vi "Settings.vi"(8 "error in (no error)":errorcluster, 9 "Gantry Region":i32=1, 11 "Assembly Tray In":refnum<class "Assembly Tray.lvclass">) -> (0 "error out":errorcluster, 3 "Assembly Tray Out":refnum<class "Assembly Tray.lvclass">)   [LabVIEW 2020, in "Assembly Tray.lvclass"]
uses:
  Assembly Tray.lvclass
panel:
  in  "Component Thickness":dbl=2.0 format="%#_13g"
  in  "Submit":bool
  in  "Position Number":i32=1
  in  "Tray Number":i32=1
  # "Assembly Tray"
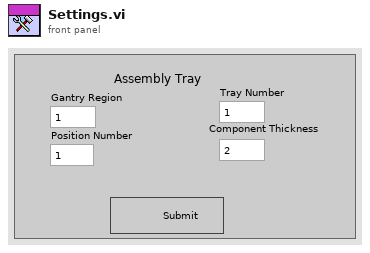
[diagram p1: front panel]
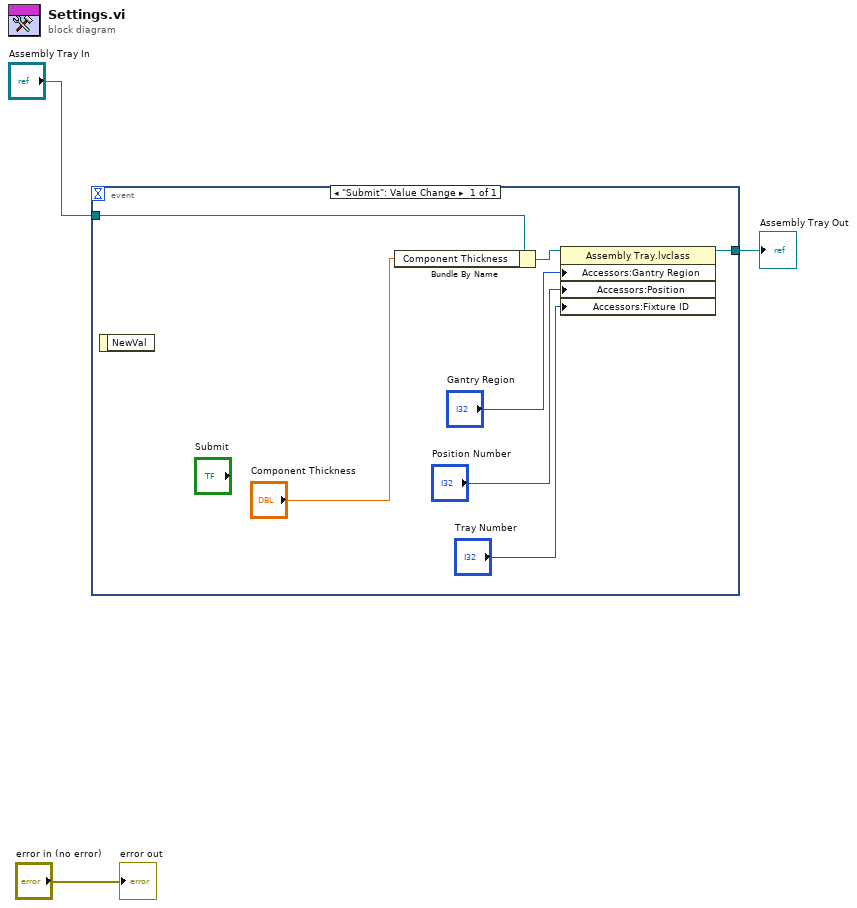
[diagram p0: block diagram]
diagram:
  n1 = event shown="[0] \"Submit\": Value Change" {
    selector: _ -> [_]
    dyn-events: _ -> [_]
    timeout: _ -> [_]
    tunnel: "Assembly Tray In" -> [w9]
    tunnel: [w6] -> w2
    event "Submit": Value Change {
      n2 = event-data() -> ()  [unwired: 1 in, 1 out]
      n3 = Bundle By Name(cluster=w9, "Component Thickness"="Component Thickness") -> (w8:refnum<class "Assembly Tray.lvclass">)
      n4 = property class="Assembly Tray.lvclass"(reference=w8, "Accessors:Gantry Region"="Gantry Region", "Accessors:Position"="Position Number", "Accessors:Fixture ID"="Tray Number") -> (reference out=w6:refnum<class "Assembly Tray.lvclass">)  [unwired: 1 in, 1 out]
    }
  }
  "Assembly Tray Out" <- w2
  "error out" <- "error in (no error)"
